vi "Withdrawal_failed.vi"(8 "error in (no error)":errorcluster, 11 "Withdrawal_failed in":refnum<class "Withdrawal_failed.lvclass">) -> (0 "error out":errorcluster, 3 "State out":refnum<class "State Actor.lvclass">)   [LabVIEW 2025, in "ATM_UI_Controller.lvlib" / "Withdrawal_failed.lvclass"]
uses:
  Withdrawal_failed.lvclass
  Withdrawal_failed.lvclass/Withdrawal_failed.ctl
  C:/Users/halstead_rideriver/Documents/Labview_Practice/ATM_Machine_Actor Framework/ATM_ACTORFW/ATM_UI_Controller/ATM_UI_Controller.lvclass
  C:/Program Files (x86)/National Instruments/LabVIEW 2025/vi.lib/ni/Actors/State Actor/State Actor/State Actor.lvclass
  C:/Program Files (x86)/National Instruments/LabVIEW 2025/vi.lib/ActorFramework/Actor/Actor.lvclass
  C:/Users/halstead_rideriver/Documents/Labview_Practice/ATM_Machine_Actor Framework/ATM_ACTORFW/ATM_UI_Controller/Withdrawal_failed/Withdrawal_failed.lvclass
  <vilib>/ni/Actors/State Actor/State Actor/State Actor.lvclass
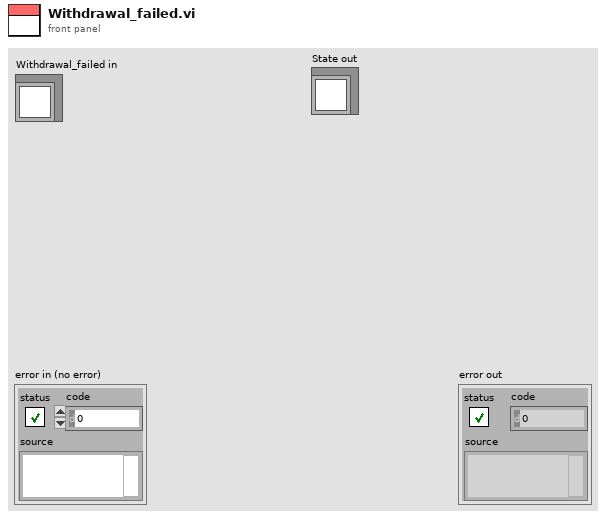
[diagram p1: front panel]
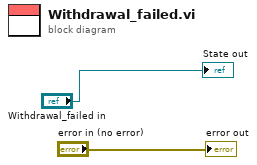
[diagram p0: block diagram]
diagram:
  "error out" <- "error in (no error)"
  "State out" <- "Withdrawal_failed in"
